vi "Import Sensors from CSV.vi"(10 "CSV Path":path=path "C:/Data/Rel Lab Gauges Slope Offset.csv", 11 "Sensors":T1[](array[typedef]) {"Max Error % of Reading" format="%.2f"; "Max Stability Error" format="%.2f"; "Max Mean Squared Error" format="%.2f"; "Max Error % of Full Scale" format="%.2f"; "Coefficients" format="%.2f"; "Voltage List" format="%.2f"; "EGU List" format="%.2f"; "EGU Range"."Low Limit" format="%.2f"; "EGU Range"."High Limit" format="%.2f"; "Voltage Range"."Low Limit" format="%.2f"; "Voltage Range"."High Limit" format="%.2f"; "Last Cal Info"."Last Calibration Date" format="%.2f"}) -> (3 "Sensors OUT":T1[](array[typedef]) {"Max Error % of Reading" format="%.2f"; "Max Stability Error" format="%.2f"; "Max Mean Squared Error" format="%.2f"; "Max Error % of Full Scale" format="%.2f"; "Coefficients" format="%.2f"; "Voltage List" format="%.2f"; "EGU List" format="%.2f"; "EGU Range"."Low Limit" format="%.2f"; "EGU Range"."High Limit" format="%.2f"; "Voltage Range"."Low Limit" format="%.2f"; "Voltage Range"."High Limit" format="%.2f"; "Last Cal Info"."Last Calibration Date" format="%.2f"})   [LabVIEW 2023]
uses:
  Type Defs and Controls/Sensor.ctl
  <vilib>/Utility/miscctls.llb/LVDateTimeRec.ctl
  <vilib>/Utility/file.llb/Read Delimited Spreadsheet (string).vi
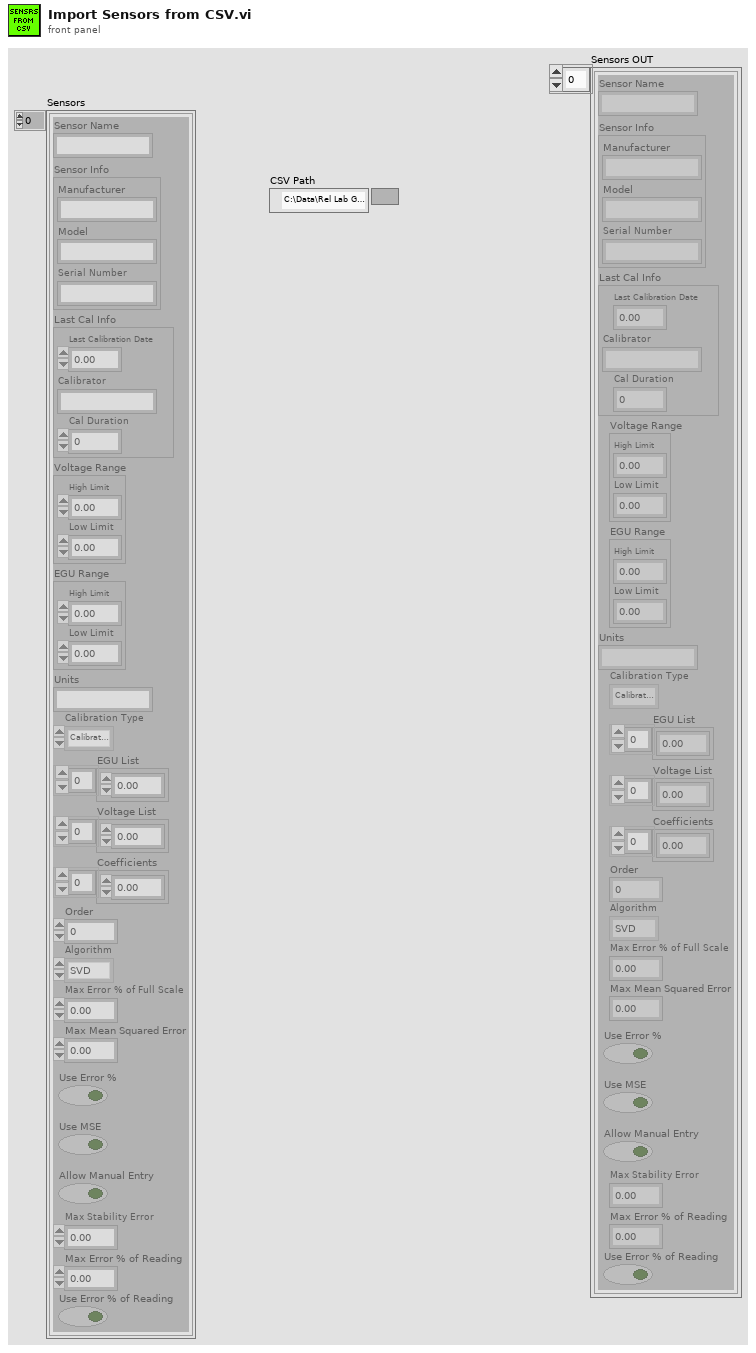
[diagram p1: front panel]
types:
  T1 = typedef "Sensor.ctl" = cluster{"Sensor Name":string, "Sensor Info":cluster{"Manufacturer":string, "Model":string, "Serial Number":string}, "Last Cal Info":cluster{"Last Calibration Date":dbl, "Calibrator":string, "Cal Duration":i32}, "Voltage Range":cluster{"High Limit":dbl, "Low Limit":dbl}, "EGU Range":cluster{"High Limit":dbl, "Low Limit":dbl}, "Units":string, "Calibration Type":enum16{"Calibrate Analog", "Compare Analog Calibration"}, "EGU List":dbl[], "Voltage List":dbl[], "Coefficients":dbl[], "Order":i32, "Algorithm":enum32{"SVD", "Givens", "Givens2", "Householder", "LU Decomposition", "Cholesky"}, "Max Error % of Full Scale":dbl, "Max Mean Squared Error":dbl, "Use Error %":bool, "Use MSE":bool, "Allow Manual Entry":bool, "Max Stability Error":dbl, "Max Error % of Reading":dbl, "Use Error % of Reading":bool}
  T2 = typedef "LVDateTimeRec.ctl" = cluster{"fractional second":dbl, "second":i32, "minute":i32, "hour":i32, "day of month":i32, "month":i32, "year":i32, "day of week":i32, "day of year":i32, "DST":i32}
  T3 = cluster{"Sensor Name":string, "Sensor Info":cluster{"Manufacturer":string, "Model":string, "Serial Number":string}, "Last Cal Info":cluster{"Last Calibration Date":dbl, "Calibrator":string, "Cal Duration":i32}, "Voltage Range":cluster{"High Limit":dbl, "Low Limit":dbl}, "EGU Range":cluster{"High Limit":dbl, "Low Limit":dbl}, "Units":string, "Calibration Type":enum16{"Calibrate Analog", "Compare Analog Calibration"}, "EGU List":dbl[], "Voltage List":dbl[], "Coefficients":dbl[], "Order":i32, "Algorithm":enum32{"SVD", "Givens", "Givens2", "Householder", "LU Decomposition", "Cholesky"}, "Max Error % of Full Scale":dbl, "Max Mean Squared Error":dbl, "Use Error %":bool, "Use MSE":bool, "Allow Manual Entry":bool, "Max Stability Error":dbl, "Max Error % of Reading":dbl, "Use Error % of Reading":bool}
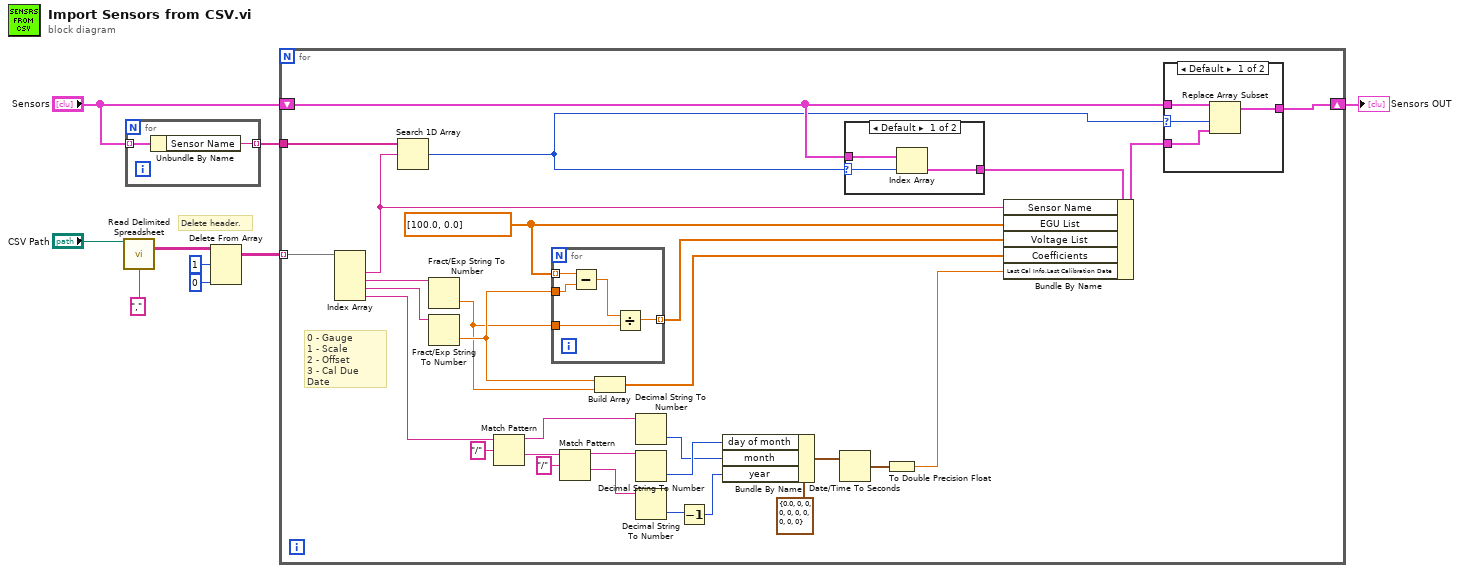
[diagram p0: block diagram]
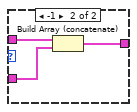
[diagram p2: hidden frame]
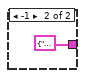
[diagram p3: hidden frame]
diagram:
  # "Delete header."
  n1 = call-poly <vilib>:"Read Delimited Spreadsheet.vi"("file path (dialog if empty)"="CSV Path", "delimiter (\\t)"="," ("delimiter (\\t)")) -> ("all rows"=w7:string[][])  [unwired: 8 in, 5 out]
  n2 = for {
    tunnel: "Sensors" -> [w11] mode=indexing
    tunnel: [w10] -> w2 mode=indexing
    n3 = Unbundle By Name(w11) -> ("Sensor Name"=w10:string)
  }
  n4 = Delete From Array(array=w7, length=1, index (row)=0) -> (array with subset deleted=w4:string[][])  [unwired: 1 in, 1 out]
  n5 = for {
    shift-right: [w40] -> w1
    shift-left: "Sensors" -> [w14]
    tunnel: w4 -> [w41] mode=indexing
    tunnel: w2 -> [w16]
    w36 = dbl[] [100.0, 0.0] ("EGU List")
    # "0 - Gauge\n1 - Scale\n2 - Offset\n3 - Cal Due Date"
    n6 = Index Array(array=w41) -> (element #1=w15:string, element #2=w38:string, element #3=w37:string, element #4=w21:string)  [unwired: 4 in]
    n7 = Search 1D Array(1D array=w16, element=w15) -> (index of element=w12:i32)  [unwired: 1 in]
    n8 = Fract/Exp String To Number(string=w38) -> (number=w33:dbl)  [unwired: 3 in, 1 out]
    n9 = Fract/Exp String To Number(string=w37) -> (number=w34:dbl)  [unwired: 3 in, 1 out]
    n10 = Match Pattern(string=w21, regular expression="/") -> (before substring=w26:string, after substring=w24:string)  [unwired: 1 in, 2 out]
    n11 = for {
      tunnel: w36 -> [w57] mode=indexing
      tunnel: [w55] -> w35 mode=indexing
      tunnel: w34 -> [w56]
      tunnel: w33 -> [w53]
      n12 = Subtract(x=w57, y=w56) -> (x-y=w54:dbl)
      n13 = Divide(x=w54, y=w53) -> (x/y=w55:dbl)
    }
    n14 = Match Pattern(string=w24, regular expression="/") -> (before substring=w28:string, after substring=w30:string)  [unwired: 1 in, 2 out]
    n15 = Build Array(w34, w33) -> (w32:dbl[])
    n16 = Decimal String To Number(string=w26) -> (number=w27:i32)  [unwired: 2 in, 1 out]
    n17 = Decimal String To Number(string=w28) -> (number=w29:i32)  [unwired: 2 in, 1 out]
    n18 = Decimal String To Number(string=w30) -> (number=w20:i32)  [unwired: 2 in, 1 out]
    n19 = Decrement(x=w20) -> (x-1=w19:i32)
    n20 = Bundle By Name(cluster=T2 {"fractional second"=0.0, "second"=0, "minute"=0, "hour"=0, "day of month"=0, "month"=0, "year"=0, "day of week"=0, "day of year"=0, "DST"=0} ("date time rec"), "day of month"=w29, "month"=w27, "year"=w19) -> (w31:T2)
    n21 = Date/Time To Seconds(2:w31) -> (0:w18:timestamp)  [unwired: 1 in]
    n22 = case shown="Default" w12 {
      selector: w12 -> [w51 _]
      tunnel: w14 -> [w50 _]
      tunnel: [w49 T3 {"Sensor Name"="", "Sensor Info"={"Manufacturer"="", "Model"="", "Serial Number"=""}, "Last Cal Info"={"Last Calibration Date"=0.0, "Calibrator"="", "Cal Duration"=0}, "Voltage Range"={"High Limit"=0.0, "Low Limit"=0.0}, "EGU Range"={"High Limit"=0.0, "Low Limit"=0.0}, "Units"="", "Calibration Type"=enum."Calibrate Analog", "EGU List"=[], "Voltage List"=[], "Coefficients"=[], "Order"=0, "Algorithm"=enum."SVD", "Max Error % of Full Scale"=0.0, "Max Mean Squared Error"=0.0, "Use Error %"=FALSE, "Use MSE"=FALSE, "Allow Manual Entry"=FALSE, "Max Stability Error"=0.0, "Max Error % of Reading"=0.0, "Use Error % of Reading"=FALSE} ("Sensor Description")] -> w13
      frame Default {
        n23 = Index Array(array=w50, index=w51) -> (element=w49:T1)
      }
      frame -1 {
      }
    }
    n24 = To Double Precision Float(number=w18) -> (double precision float=w17:dbl)
    n25 = Bundle By Name(cluster=w13, "Sensor Name"=w15, "EGU List"=w36, "Voltage List"=w35, "Coefficients"=w32, "Last Cal Info.Last Calibration Date"=w17) -> (w39:T1)
    n26 = case shown="Default" w12 {
      selector: w12 -> [w43 _]
      tunnel: [w44 w48] -> w40
      tunnel: w39 -> [w42 w47]
      tunnel: w14 -> [w45 w46]
      frame Default {
        n27 = Replace Array Subset(array=w45, new element=w42, index=w43) -> (w44:T1[])
      }
      frame -1 {
        n28 = Build Array (concatenate)(w46, w47) -> (w48:T1[])
      }
    }
  }
  "Sensors OUT" <- w1
